vi "LoopSetStopCondition.vi"(8 "ErrorArray":errorcluster[](array[cluster]), 9 "StopCondition":variant, 11 "Test.lvclass":refnum<class "Test.lvclass">) -> (0 "ErrorArray":errorcluster[](array[cluster]), 3 "Test.lvclass":refnum<class "Test.lvclass">)   [LabVIEW 2018, in "Test.lvclass"]
uses:
  Test.lvclass
  Test.lvclass/Test.ctl
  Accessors/Read LoopStopCondition.vi
  Accessors/Write LoopStopCondition.vi
  Accessors/Read ErrorSeverity.vi
  <vilib>/Utility/error.llb/Error Cluster From Error Code.vi
  <vilib>/ErrorRing/Error Ring.xnode
  <userlib>/NIST/NISTErrorLib/NISTErrorLib.lvlib
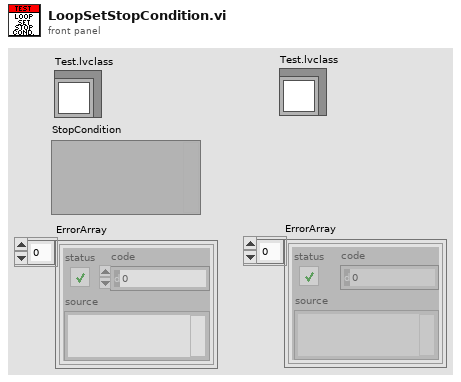
[diagram p1: front panel]
types:
  T1 = typedef "Test.lvclass/LoopStopCondition.ctl" = cluster{"Name":string, "StopCondition":variant}
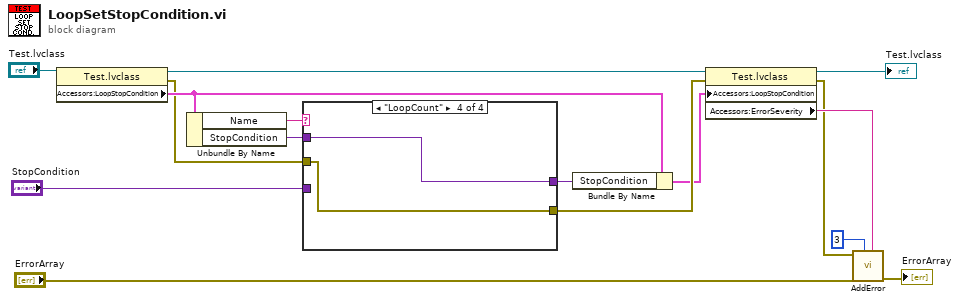
[diagram p0: block diagram]
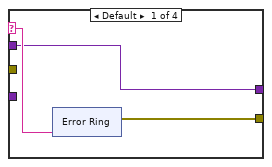
[diagram p2: hidden frame]
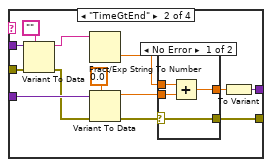
[diagram p3: hidden frame]
diagram:
  n1 = property class="Test.lvclass"(reference="Test.lvclass") -> (reference out=w6:refnum<class "Test.lvclass">, error out=w10:errorcluster, "Accessors:LoopStopCondition"=w12:T1)  [unwired: 1 in]
  n2 = Unbundle By Name(w12) -> ("Name"=w15:string, "StopCondition"=w13:variant)
  n3 = case shown="\"LoopCount\"" w15 {
    selector: w15 -> [w19 _ _ _]
    tunnel: "StopCondition" -> [_ w38 _ _]
    tunnel: w13 -> [w17 w39 w46 w48]
    tunnel: [w18 w33 w45 w47] -> w7
    tunnel: [w17 w31 w46 w48] -> w11
    tunnel: w10 -> [_ w35 w45 w47]
    frame Default {
      n4 = xnode "Error Ring"("parameter 0"=w19) -> ("error out"=w18:errorcluster)
    }
    frame "TimeGtEnd" {
      n5 = Variant To Data(error in=w35, type="", Variant=w39) -> (data=w28:string, error out=w29:errorcluster)
      n6 = Fract/Exp String To Number(string=w28) -> (number=w27:dbl)  [unwired: 3 in, 1 out]
      n7 = Variant To Data(error in=w29, type=0.0, Variant=w38) -> (data=w36:dbl, error out=w34:errorcluster)
      n8 = case shown="No Error" w34 {
        selector: w34 -> [w41 _]
        tunnel: w36 -> [w43 _]
        tunnel: w27 -> [w42 w44]
        tunnel: [w40 w44] -> w32
        tunnel: [w41 _] -> w33
        frame No Error {
          n9 = Add(x=w42, y=w43) -> (x+y=w40:dbl)
        }
        frame Error {
        }
      }
      n10 = To Variant(anything=w32) -> (Variant=w31:variant)
    }
    frame "AnalysisIdle" {
    }
    frame "LoopCount" {
    }
  }
  n11 = Bundle By Name(cluster=w12, "StopCondition"=w11) -> (w5:T1)
  n12 = property class="Test.lvclass"(reference=w6, error in=w7, "Accessors:LoopStopCondition"=w5) -> (reference out=→"Test.lvclass":refnum<class "Test.lvclass">, error out=w1:errorcluster, "Accessors:ErrorSeverity"=w4:string)
  n13 = call <userlib>:"AddError.vi"("Severity"=w4, "Priority"=u8 3, "ErrorArray In"="ErrorArray", "error in (no error)"=w1) -> ("ErrorArray Out"=→"ErrorArray":errorcluster[])  [unwired: 6 in, 1 out]
